vi "GetPointType4D_2D-DBL.vi"(11 "Point":T2) -> (3 "Point":T1)   [LabVIEW 2020, in "OpenLvVision_OpenCv.lvlib"]
uses:
  OpenLvVision_OpenCv.lvlib
  TypeDef/Point/4D_PointDBL.ctl
  TypeDef/Point/2D_PointDBL.ctl
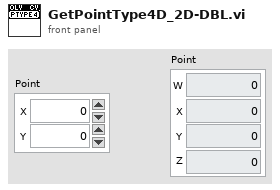
[diagram p1: front panel]
types:
  T1 = typedef "OpenLvVision_OpenCv.lvlib/4D_PointDBL.ctl" = cluster{"W":dbl, "X":dbl, "Y":dbl, "Z":dbl}
  T2 = typedef "OpenLvVision_OpenCv.lvlib/2D_PointDBL.ctl" = cluster{"X":dbl, "Y":dbl}
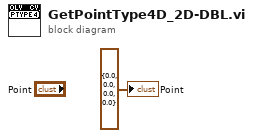
[diagram p0: block diagram]
diagram:
  "Point" <- T1 {"W"=0.0, "X"=0.0, "Y"=0.0, "Z"=0.0} ("Point")
